vi "Stop_Action.vi"(8 "error in (no error)":errorcluster caption="错误输入（无错误）") -> (0 "error out":errorcluster caption="错误输出")   [LabVIEW 2013]
uses:
  InstrumentDrivers/USB-CAN/DevType.ctl
  <resource>/objmgr/daqmx.rc
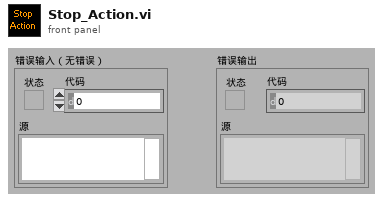
[diagram p1: front panel]
types:
  T1 = typedef "DevType.ctl" = u16
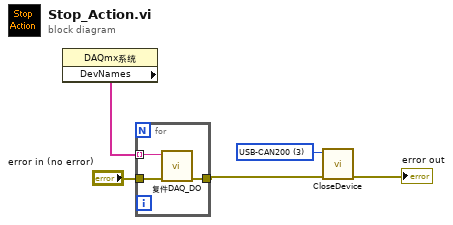
[diagram p0: block diagram]
diagram:
  w1 = T1 3 items=["PCI-CAN200"=7, "USB-CAN"=2, "USB-CAN200"=3] ("DeviceType")
  n1 = property class="DAQmx系统"() -> ("DevNames"=w4:tag[])  [unwired: 2 in, 2 out]
  n2 = for {
    tunnel: [w8] -> w3
    tunnel: "error in (no error)" -> [w7]
    tunnel: w4 -> [w6] mode=indexing
    n3 = call "复件DAQ_DO.vi"("error in"=w7, "device in"=w6) -> ("error out"=w8:errorcluster)  [unwired: 9 in]
  }
  n4 = call "CloseDevice.vi"("错误输入（无错误）"=w3, "DeviceType"=w1) -> ("错误输出"=→"error out":errorcluster)  [unwired: 7 in, 2 out]
